vi "CRYUnary Curve.vi"(0 "Operand A":T2={"Name"="", "Curve"=[], "X data"=1, "Y data"=1, "Z data"=1, "X axis"=0, "Y axis"=1, "Z axis"=1, "X unit"="Hz", "Y unit"="", "Z unit"="deg.", "X dB ref"=1.0, "Y dB ref"=1.0, "Z dB ref"=1.0, "single val"=FALSE, "protected"=FALSE, "display X"=TRUE, "display Y"=TRUE, "display Z"=TRUE, "Test Info"="", "Step No."=0, "Plot Settings"={"Color"=0, "Interpolation"=0, "Point Style"=0, "Line Style"=0, "Point Color"=0, "Line Width"=0, "Bar Plot Style"=0, "Fill To"=0}, "AutoProtect"=FALSE} {"Z data" items=["dB", "Lin"]; "X data" items=["dB", "Lin"]; "Y data" items=["dB", "Lin"]; "Z dB ref" format="%.1f"; "Z axis" items=["Log", "Lin"]; "X dB ref" format="%.1f"; "X axis" items=["Log", "Lin"]; "Y axis" items=["Log", "Lin"]; "Y dB ref" format="%.1f"; "Curve"."z" format="%.2f"; "Curve"."y" format="%.2f"; "Curve"."x" format="%.2f"}, 1 "Type A":enum16{"Curves", "Values", "Results", "WFM"}(ring), 2 "All points":bool, 5 "A _axis mode":u16(slide) scale=0.0..2.0, 7 "Unary Operator":u16(ring) items=["Change Sign", "Reciprocal Value", "Absolute Value", "Square", "Square Root", "Exp", "Ln", "Unwarp Phase", "Group Delay", "FFT", "Inverse FFT"], 9 "Wave in":T1={"Waveform"={"X0"=0.0, "dX"=0.0, "Y"=[]}, "X data"=1, "Y data"=1, "Y axis"=1, "X unit"="s", "Y unit"="V", "Y dB ref"=1.0, "display Y"=TRUE, "display X"=TRUE, "Overload?"=FALSE, "Test Info"="", "Step No."=0, "Name"="", "protected"=FALSE, "Sqc history"=[], "Signal Channel ID"=0, "Plot Settings"={"Color"=0, "Interpolation"=0, "Point Style"=0, "Line Style"=0, "Point Color"=0, "Line Width"=0, "Bar Plot Style"=0, "Fill To"=0}, "AutoProtect"=FALSE} {"Y dB ref" format="%.1f"; "Y axis" items=["Log", "Lin"]; "Y data" items=["dB", "Lin"]; "X data" items=["dB", "Lin"]}, 11 "Search Items":string[](array[string]), 12 "Win Mode":u16(ring) items=["None", "Cosine Traper", "Exponential"], 13 "Smoothing Width":i32, 14 "Sampling Rate":dbl) -> (4 "Result":T2={"Name"="", "Curve"=[], "X data"=1, "Y data"=1, "Z data"=1, "X axis"=0, "Y axis"=1, "Z axis"=1, "X unit"="Hz", "Y unit"="", "Z unit"="deg.", "X dB ref"=1.0, "Y dB ref"=1.0, "Z dB ref"=1.0, "single val"=FALSE, "protected"=FALSE, "display X"=TRUE, "display Y"=TRUE, "display Z"=TRUE, "Test Info"="", "Step No."=0, "Plot Settings"={"Color"=0, "Interpolation"=0, "Point Style"=0, "Line Style"=0, "Point Color"=0, "Line Width"=0, "Bar Plot Style"=0, "Fill To"=0}, "AutoProtect"=FALSE} {"Z data" items=["dB", "Lin"]; "X data" items=["dB", "Lin"]; "Y data" items=["dB", "Lin"]; "Z dB ref" format="%.1f"; "Z axis" items=["Log", "Lin"]; "X dB ref" format="%.1f"; "X axis" items=["Log", "Lin"]; "Y axis" items=["Log", "Lin"]; "Y dB ref" format="%.1f"; "Curve"."z" format="%.2f"; "Curve"."y" format="%.2f"; "Curve"."x" format="%.2f"}, 6 "Type out":enum16{"Curves", "Values", "Results", "WFM"}(ring), 10 "Wave out":T1={"Waveform"={"X0"=0.0, "dX"=0.0, "Y"=[]}, "X data"=1, "Y data"=1, "Y axis"=1, "X unit"="s", "Y unit"="V", "Y dB ref"=1.0, "display Y"=TRUE, "display X"=TRUE, "Overload?"=FALSE, "Test Info"="", "Step No."=0, "Name"="", "protected"=FALSE, "Sqc history"=[], "Signal Channel ID"=0, "Plot Settings"={"Color"=0, "Interpolation"=0, "Point Style"=0, "Line Style"=0, "Point Color"=0, "Line Width"=0, "Bar Plot Style"=0, "Fill To"=0}, "AutoProtect"=FALSE} {"Y dB ref" format="%.1f"; "Y axis" items=["Log", "Lin"]; "Y data" items=["dB", "Lin"]; "X data" items=["dB", "Lin"]})   [LabVIEW 2013]
uses:
  Typedef Control/CRYData Cluster.ctl
  Typedef Control/CRYWaveform Cluster.ctl
  <vilib>/Analysis/4window.llb/Cosine Tapered Window (CDB).vi
  <vilib>/Analysis/4window.llb/Exponential Window (CDB).vi
  <vilib>/Analysis/2dsp.llb/Complex FFT.vi
  <vilib>/Analysis/2dsp.llb/Inverse Real FFT.vi
  CRYPost Processing Global.vi
  <vilib>/Analysis/NI_AALPro.lvlib
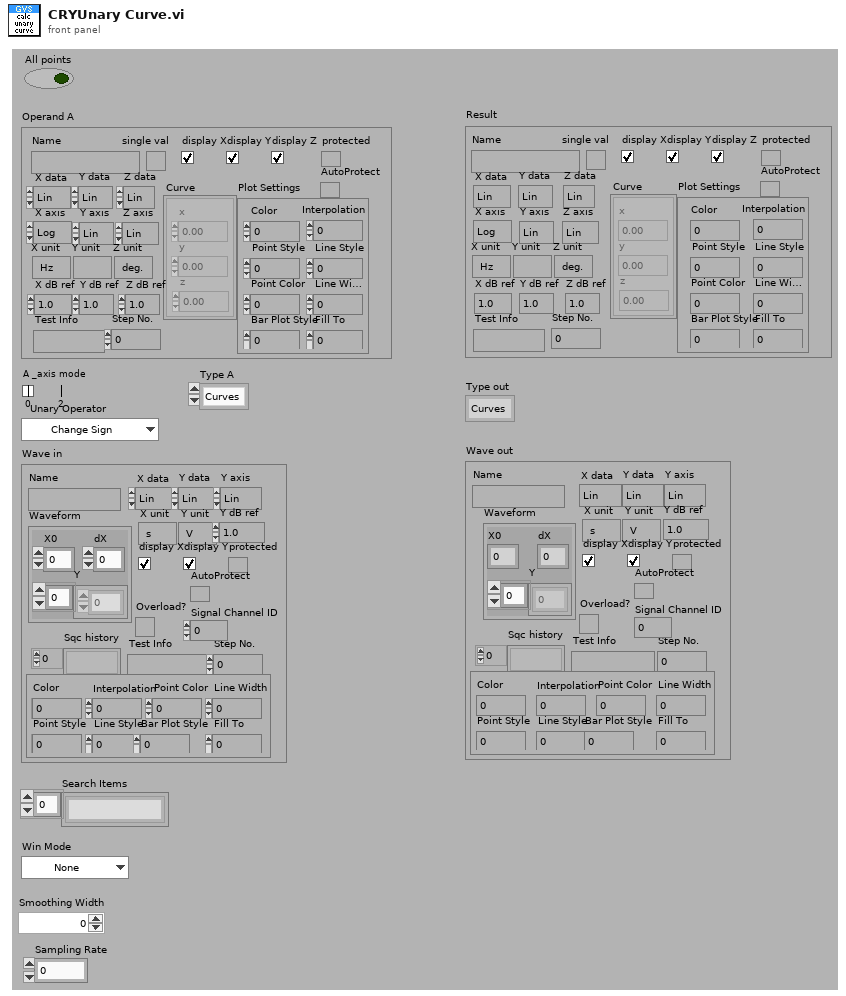
[diagram p1: front panel]
types:
  T1 = typedef "CRYWaveform Cluster.ctl" = cluster{"Waveform":cluster{"X0":dbl, "dX":dbl, "Y":sgl[]}, "X data":u16, "Y data":u16, "Y axis":u16, "X unit":string, "Y unit":string, "Y dB ref":dbl, "display Y":bool, "display X":bool, "Overload?":bool, "Test Info":string, "Step No.":i32, "Name":string, "protected":bool, "Sqc history":string[], "Signal Channel ID":i32, "Plot Settings":cluster{"Color":u32, "Interpolation":u8, "Point Style":u8, "Line Style":u8, "Point Color":u32, "Line Width":u8, "Bar Plot Style":u8, "Fill To":i16}, "AutoProtect":bool}
  T2 = typedef "CRYData Cluster.ctl" = cluster{"Name":string, "Curve":cluster{"x":dbl, "y":dbl, "z":dbl}[], "X data":u16, "Y data":u16, "Z data":u16, "X axis":u16, "Y axis":u16, "Z axis":u16, "X unit":string, "Y unit":string, "Z unit":string, "X dB ref":dbl, "Y dB ref":dbl, "Z dB ref":dbl, "single val":bool, "protected":bool, "display X":bool, "display Y":bool, "display Z":bool, "Test Info":string, "Step No.":i32, "Plot Settings":cluster{"Color":u32, "Interpolation":u8, "Point Style":u8, "Line Style":u8, "Point Color":u32, "Line Width":u8, "Bar Plot Style":u8, "Fill To":i16}, "AutoProtect":bool}
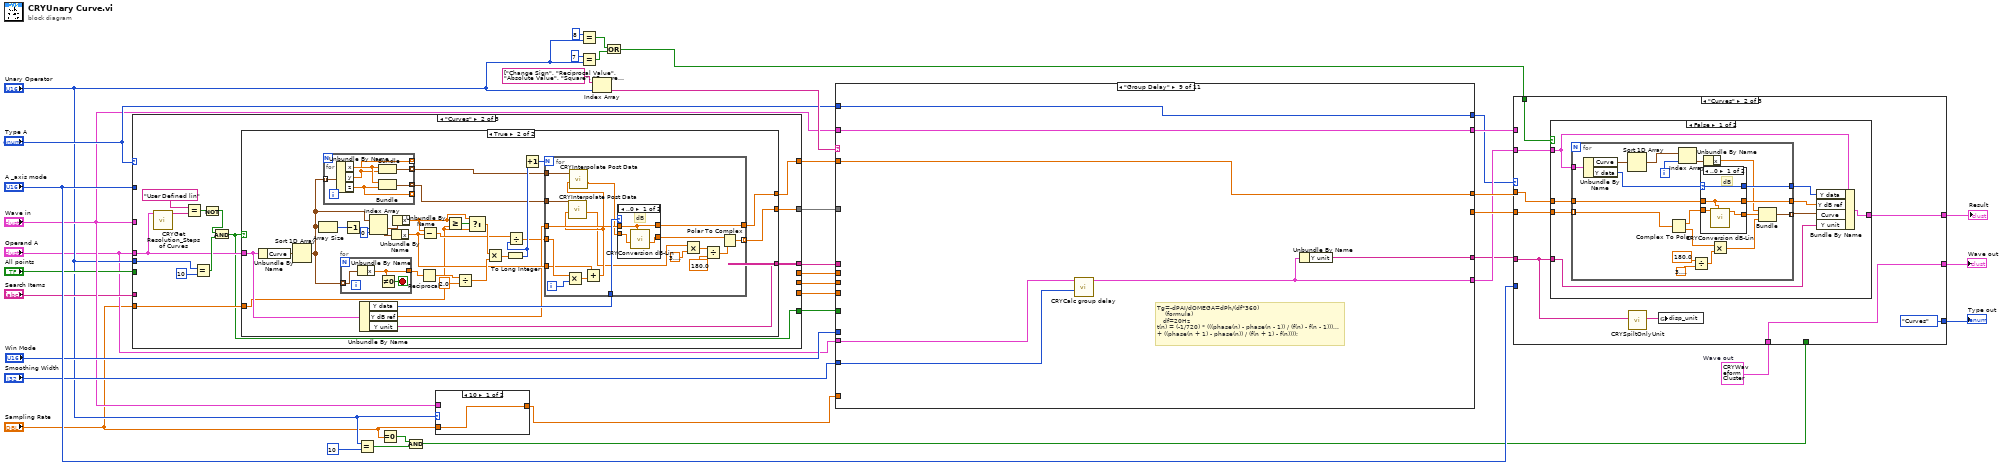
[diagram p0: block diagram]
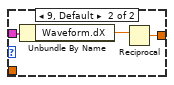
[diagram p2: hidden frame]
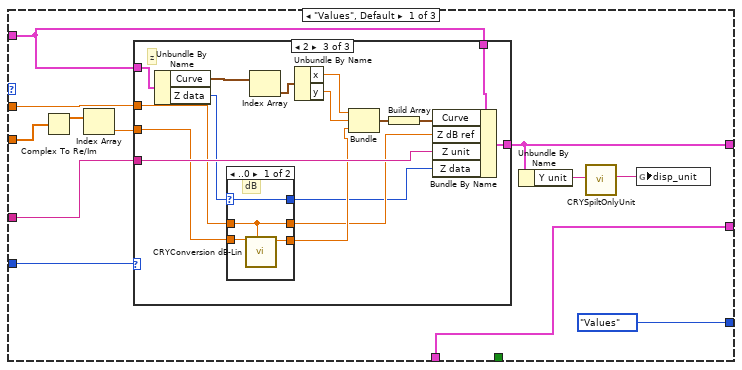
[diagram p3: hidden frame]
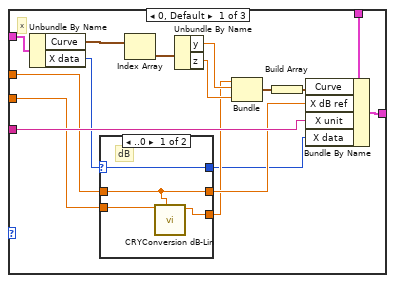
[diagram p4: hidden frame]
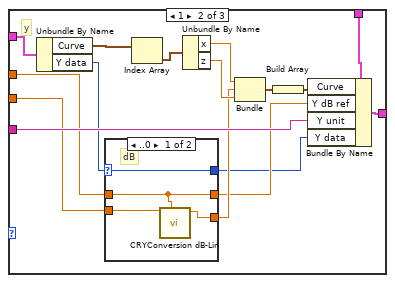
[diagram p6: hidden frame]
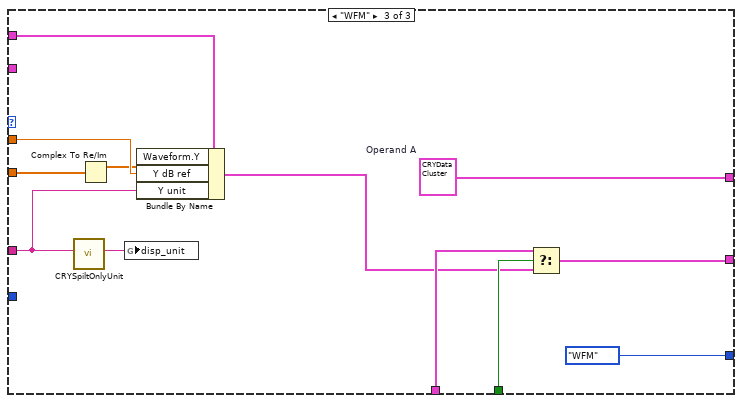
[diagram p11: hidden frame]
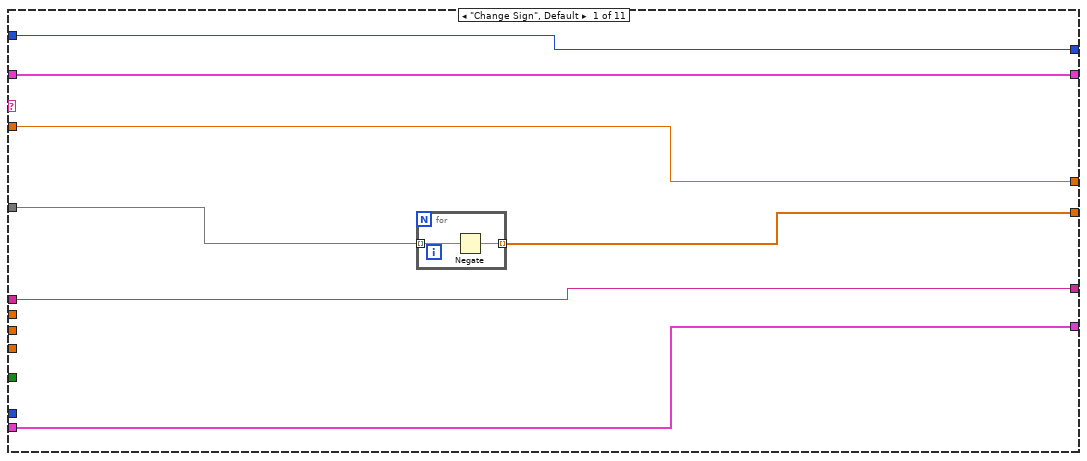
[diagram p12: hidden frame]
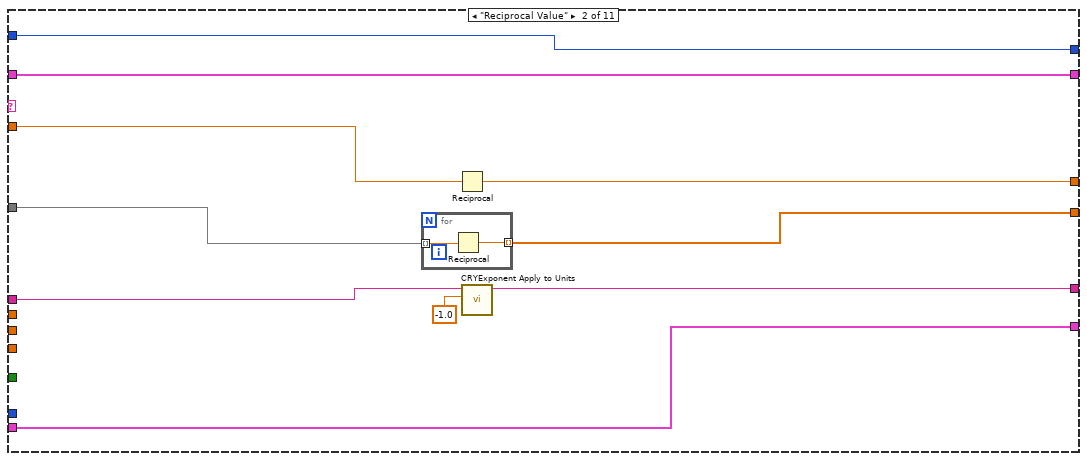
[diagram p13: hidden frame]
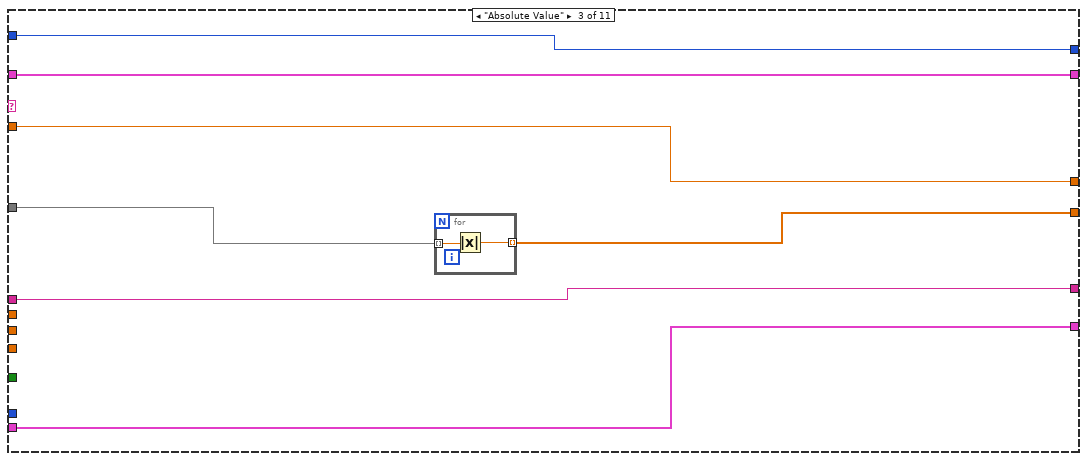
[diagram p14: hidden frame]
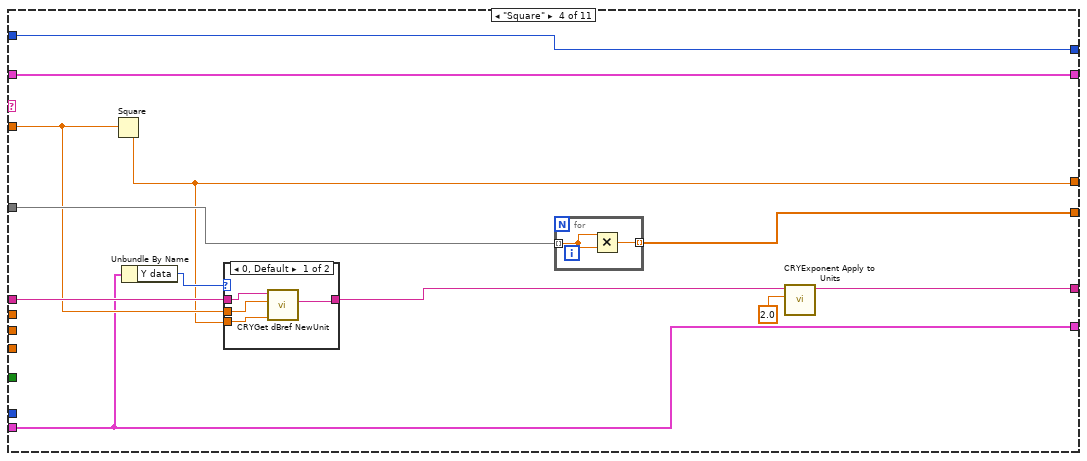
[diagram p15: hidden frame]
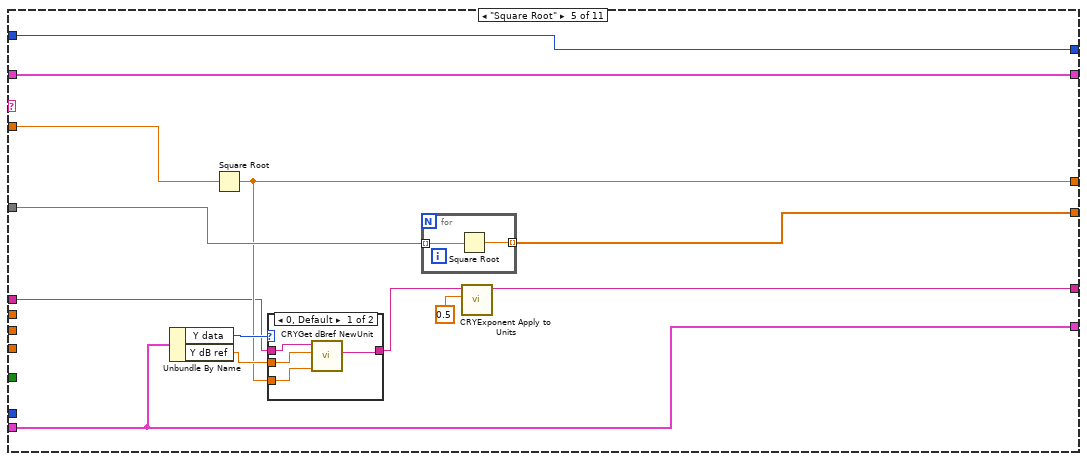
[diagram p17: hidden frame]
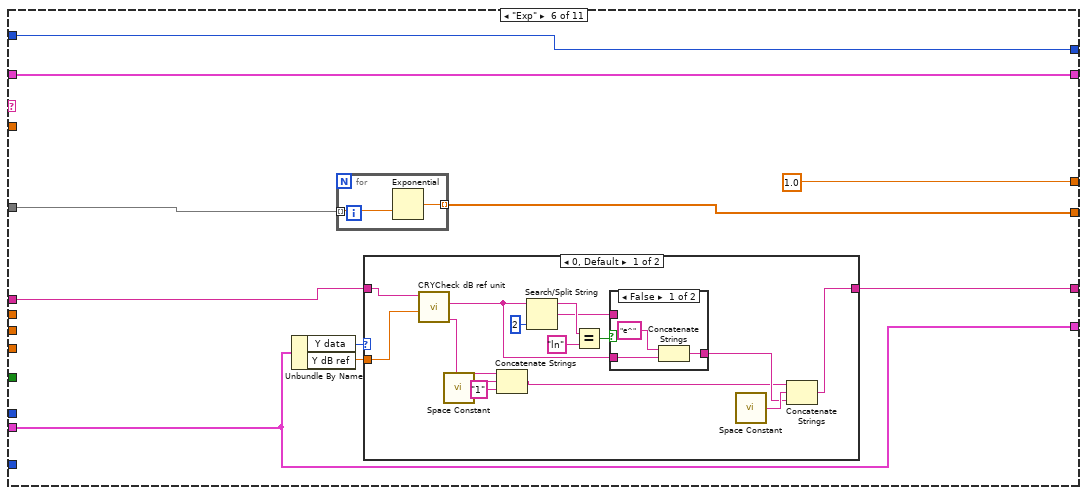
[diagram p19: hidden frame]
diagram:
  w5 = T1 {"Waveform"={"X0"=0.0, "dX"=0.0, "Y"=[]}, "X data"=1, "Y data"=1, "Y axis"=1, "X unit"="s", "Y unit"="V", "Y dB ref"=1.0, "display Y"=TRUE, "display X"=TRUE, "Overload?"=FALSE, "Test Info"="", "Step No."=0, "Name"="", "protected"=FALSE, "Sqc history"=[], "Signal Channel ID"=0, "Plot Settings"={"Color"=0, "Interpolation"=0, "Point Style"=0, "Line Style"=0, "Point Color"=0, "Line Width"=0, "Bar Plot Style"=0, "Fill To"=0}, "AutoProtect"=FALSE}  # Wave out
  n1 = case shown="\"Curves\"" "Type A" {
    tunnel: [w47 w100 w193] -> w12
    tunnel: [w46 w102 w201] -> w36
    tunnel: [w43 w101 w202] -> w37
    tunnel: "Operand A" -> [w44 w91 _]
    tunnel: "A _axis mode" -> [w45 _ _]
    tunnel: "Wave in" -> [_ _ w203]
    tunnel: "Search Items" -> [_ _ w196]
    tunnel: "All points" -> [_ _ w200]
    tunnel: [_ _ w195] -> w15
    tunnel: [_ _ w194] -> w14
    tunnel: [_ _ w192] -> w13
    tunnel: "Unary Operator" -> [_ w94 w191]
    tunnel: "Sampling Rate" -> [_ w99 _]
    tunnel: [_ w90 _] -> w2
    frame "Values", Default {
      n2 = case shown="0, Default" w45 {
        tunnel: w44 -> [w56 w68 w82]
        tunnel: [w48 w63 w76] -> w42
        tunnel: [w53 w67 w81] -> w46
        tunnel: [w49 w62 w77] -> w43
        frame 0, Default {
          # "x"
          n3 = Unbundle By Name(w56) -> ("X data"=w52:u16, "X dB ref"=w51:dbl, "Curve"=w55:cluster{"x":dbl, "y":dbl, "z":dbl}[], "X unit"=w53:string)
          n4 = Index Array(array=w55) -> (element=w54:cluster{"x":dbl, "y":dbl, "z":dbl})  [unwired: 1 in]
          n5 = Unbundle By Name(w54) -> ("x"=w50:dbl)
          n6 = case shown="1.." w52 {
            tunnel: w50 -> [w57 w61]
            tunnel: [w59 w61] -> w48
            tunnel: w51 -> [w58 w60]
            tunnel: [w58 w60] -> w49
            frame ..0 {
              # "dB"
              n7 = call "CRYConversion dB-Lin.vi"("dB ref."=w58, "Log In"=w57) -> ("Lin Out"=w59:dbl)  [unwired: 4 in, 3 out]
            }
            frame 1.. {
            }
          }
        }
        frame 1 {
          # "y"
          n8 = Unbundle By Name(w68) -> ("Y data"=w66:u16, "Y dB ref"=w64:dbl, "Curve"=w70:cluster{"x":dbl, "y":dbl, "z":dbl}[], "Y unit"=w67:string)
          n9 = Index Array(array=w70) -> (element=w69:cluster{"x":dbl, "y":dbl, "z":dbl})  [unwired: 1 in]
          n10 = Unbundle By Name(w69) -> ("y"=w65:dbl)
          n11 = case shown="1.." w66 {
            tunnel: w65 -> [w73 w75]
            tunnel: [w72 w75] -> w63
            tunnel: w64 -> [w71 w74]
            tunnel: [w71 w74] -> w62
            frame ..0 {
              # "dB"
              n12 = call "CRYConversion dB-Lin.vi"("dB ref."=w71, "Log In"=w73) -> ("Lin Out"=w72:dbl)  [unwired: 4 in, 3 out]
            }
            frame 1.. {
            }
          }
        }
        frame 2 {
          # "Z"
          n13 = Unbundle By Name(w82) -> ("Z data"=w80:u16, "Z dB ref"=w79:dbl, "Curve"=w84:cluster{"x":dbl, "y":dbl, "z":dbl}[], "Z unit"=w81:string)
          n14 = Index Array(array=w84) -> (element=w83:cluster{"x":dbl, "y":dbl, "z":dbl})  [unwired: 1 in]
          n15 = Unbundle By Name(w83) -> ("z"=w78:dbl)
          n16 = case shown="..0" w80 {
            tunnel: w78 -> [w86 w89]
            tunnel: [w87 w89] -> w76
            tunnel: w79 -> [w85 w88]
            tunnel: [w85 w88] -> w77
            frame ..0 {
              # "dB"
              n17 = call "CRYConversion dB-Lin.vi"("dB ref."=w85, "Log In"=w86) -> ("Lin Out"=w87:dbl)  [unwired: 4 in, 3 out]
            }
            frame 1.. {
            }
          }
        }
      }
      n18 = Polar To Complex(1:0.0 ("theta"), 2:w42) -> (0:w41:cdb)
      n19 = Build Array(w41) -> (w47:cdb[])
    }
    frame "Curves" {
      n20 = call "CRYGet Resolution_Steps of Curves.vi"("Curve In"=w91) -> ("Original Resolution Out"=w98:string)  [unwired: 9 in, 1 out]
      n21 = Equal?(x="User Defined lin", y=w98) -> (x = y?=w96:bool)
      n22 = Equal?(x=w94, y=u16 10) -> (x = y?=w92:bool)
      n23 = Not(x=w96) -> (.not. x?=w93:bool)
      n24 = And(x=w93, y=w92) -> (x .and. y?=w90:bool)
      n25 = case shown="True" w90 {
        tunnel: w91 -> [w110 w132]
        tunnel: [w109 w128] -> w102
        tunnel: [w108 w130] -> w101
        tunnel: [w107 w129] -> w100
        tunnel: w99 -> [_ w131]
        frame False {
          n26 = Unbundle By Name(w110) -> ("Y data"=w105:u16, "Y dB ref"=w104:dbl, "Curve"=w106:cluster{"x":dbl, "y":dbl, "z":dbl}[], "Y unit"=w109:string)
          n27 = Sort 1D Array(array=w106) -> (sorted array=w103:cluster{"x":dbl, "y":dbl, "z":dbl}[])
          n28 = for {
            tunnel: w103 -> [w122] mode=indexing
            tunnel: [w121] -> w107 mode=indexing
            tunnel: w105 -> [w120]
            tunnel: w104 -> [w113]
            tunnel: [w112] -> w108
            n29 = Unbundle By Name(w122) -> ("y"=w119:dbl, "z"=w114:dbl)  [unwired: 1 out]
            n30 = case shown="..0" w120 {
              tunnel: w119 -> [w124 w127]
              tunnel: [w125 w127] -> w111
              tunnel: w113 -> [w123 w126]
              tunnel: [w123 w126] -> w112
              frame ..0 {
                # "dB"
                n31 = call "CRYConversion dB-Lin.vi"("dB ref."=w123, "Log In"=w124) -> ("Lin Out"=w125:dbl)  [unwired: 4 in, 3 out]
              }
              frame 1.. {
              }
            }
            n32 = Multiply(x=w114, y=3.141592653589793) -> (x*y=w117:dbl)
            n33 = Divide(x=w117, y=180.0) -> (x/y=w118:dbl)
            n34 = Polar To Complex(1:w118, 2:w111) -> (0:w121:cdb)
          }
        }
        frame True {
          n35 = Unbundle By Name(w132) -> ("Curve"=w149:cluster{"x":dbl, "y":dbl, "z":dbl}[])
          n36 = Sort 1D Array(array=w149) -> (sorted array=w138:cluster{"x":dbl, "y":dbl, "z":dbl}[])
          n37 = Array Size(array=w138) -> (size(s)=w151:i32)
          n38 = for {
            tunnel: w138 -> [w165] mode=indexing
            tunnel: [w163] -> w137 mode=indexing
            tunnel: [w162] -> w136 mode=indexing
            tunnel: [w161] -> _ mode=indexing
            tunnel: [w160] -> _ mode=indexing
            n39 = Unbundle By Name(w165) -> ("x"=w164:dbl, "y"=w160:dbl, "z"=w161:dbl)
            n40 = Bundle("x"=w164, "y"=w160) -> (w163:cluster{"x":dbl, "y":dbl})  [unwired: 1 in]
            n41 = Bundle("x"=w164, "z"=w161) -> (w162:cluster{"x":dbl, "z":dbl})  [unwired: 1 in]
          }
          n42 = for {
            tunnel: w138 -> [w159] mode=indexing
            tunnel: [w157] -> w153
            stop <- w158 stop-if-true
            n43 = Unbundle By Name(w159) -> ("x"=w157:dbl)
            n44 = Not Equal To 0?(x=w157) -> (x != 0?=w158:bool)
          }
          n45 = Decrement(x=w151) -> (x-1=w150:i32)
          n46 = Unbundle By Name(w132) -> ("Y data"=w135:u16, "Y dB ref"=w134:dbl, "Y unit"=w128:string)
          n47 = Index Array(array=w138, index #1=w150, index #2=0 ("index")) -> (element #1=w152:cluster{"x":dbl, "y":dbl, "z":dbl}, element #2=w144:cluster{"x":dbl, "y":dbl, "z":dbl})
          n48 = Unbundle By Name(w144) -> ("x"=w139:dbl)
          n49 = Unbundle By Name(w152) -> ("x"=w143:dbl)
          n50 = Reciprocal(x=w153) -> (1/x=w148:dbl)
          n51 = Subtract(x=w143, y=w139) -> (x-y=w141:dbl)
          n52 = Greater Or Equal?(x=w143, y=w131) -> (x >= y?=w154:bool)
          n53 = Divide(x=w148, y=2.0) -> (x/y=w146:dbl)
          n54 = Select(t=w143, s=w154, f=w131) -> (s? t:f=w156:dbl)
          n55 = Multiply(x=w156, y=w146) -> (x*y=w155:dbl)
          n56 = To Long Integer(number=w155) -> (32bit integer=w140:i32)
          n57 = Divide(x=w141, y=w140) -> (x/y=w133:dbl)
          n58 = Increment(x=w140) -> (x+1=w142:i32)
          n59 = for {
            N: w142 -> [_]
            tunnel: w133 -> [w183]
            tunnel: w139 -> [w180]
            tunnel: w137 -> [w179]
            tunnel: w136 -> [w178]
            tunnel: w135 -> [w172]
            tunnel: w134 -> [w171]
            tunnel: [w170] -> w129 mode=indexing
            tunnel: [w169] -> w130
            i -> [w182]
            n60 = Multiply(x=w183, y=w182) -> (x*y=w181:dbl)
            n61 = Add(x=w180, y=w181) -> (x+y=w168:dbl)
            n62 = call "CRYInterpolate Post Data.vi"("X value"=w168, "Curve in"=w178) -> ("Y value"=w166:dbl)  [unwired: 9 in]
            n63 = call "CRYInterpolate Post Data.vi"("X value"=w168, "Curve in"=w179) -> ("Y value"=w167:dbl)  [unwired: 9 in]
            n64 = case shown="..0" w172 {
              tunnel: w167 -> [w185 w188]
              tunnel: [w186 w188] -> w173
              tunnel: w171 -> [w184 w187]
              tunnel: [w184 w187] -> w169
              frame ..0 {
                # "dB"
                n65 = call "CRYConversion dB-Lin.vi"("dB ref."=w184, "Log In"=w185) -> ("Lin Out"=w186:dbl)  [unwired: 4 in, 3 out]
              }
              frame 1.. {
              }
            }
            n66 = Multiply(x=w166, y=3.141592653589793) -> (x*y=w176:dbl)
            n67 = Divide(x=w176, y=180.0) -> (x/y=w177:dbl)
            n68 = Polar To Complex(1:w177, 2:w173) -> (0:w170:cdb)
          }
        }
      }
    }
    frame "WFM" {
      # "max"
      # "min"
      n69 = Unbundle By Name(w203) -> ("Y dB ref"=w202:dbl, "Waveform.Y"=w198:sgl[], "Y unit"=w201:string, "Waveform.X0"=w199:dbl, "Waveform.dX"=w197:dbl)
      n70 = Equal?(x=u16 9, y=w191) -> (x = y?=w189:bool)
      n71 = case shown="True" w189 {
        tunnel: w200 -> [_ w213]
        tunnel: w199 -> [_ w212]
        tunnel: w198 -> [w204 w211]
        tunnel: w197 -> [_ w210]
        tunnel: w196 -> [_ w209]
        tunnel: [_ w208] -> w195
        tunnel: [_ w207] -> w194
        tunnel: [w204 w206] -> w193
        tunnel: [_ w205] -> w192
        frame False {
        }
        frame True {
          n72 = case shown="False" w213 {
            tunnel: [w221 w235] -> w207
            tunnel: [w222 w238] -> w208
            tunnel: w212 -> [w225 w235]
            tunnel: w211 -> [w218 w236]
            tunnel: w210 -> [w220 w237]
            tunnel: w209 -> [w227 _]
            tunnel: [w215 w236] -> w206
            tunnel: [w214 w234] -> w205
            frame False {
              w228 = "%#p" ("format string")
              n73 = Index Array(array=w227) -> (element=w226:string)  [unwired: 1 in]
              n74 = Match Pattern(string=w226, regular expression="\\.\\.\\.") -> (before substring=w232:string, after substring=w231:string)  [unwired: 3 out]
              n75 = Scan Value(string=w231, format string=w228) -> (value=w229:dbl)  [unwired: 1 in, 1 out]
              n76 = Scan Value(string=w232, format string=w228) -> (value=w230:dbl)  [unwired: 1 in, 1 out]
              n77 = Max & Min(x=w230, y=w229) -> (max(x,y)=w222:dbl, min(x,y)=w221:dbl)
              n78 = Subtract(x=w221, y=w225) -> (x-y=w224:dbl)
              n79 = Divide(x=w224, y=w220) -> (x/y=w223:dbl)
              n80 = Subtract(x=w222, y=w221) -> (x-y=w214:dbl)
              n81 = To Long Integer(number=w223) -> (32bit integer=w217:i32)
              n82 = Divide(x=w214, y=w220) -> (x/y=w219:dbl)
              n83 = To Long Integer(number=w219) -> (32bit integer=w216:i32)
              n84 = Array Subset(array=w218, index=w217, length=w216) -> (w215:sgl[])
            }
            frame True {
              n85 = Array Size(array=w236) -> (size(s)=w239:i32)
              n86 = Multiply(x=w237, y=w239) -> (x*y=w234:dbl)
              n87 = Add(x=w235, y=w234) -> (x+y=w238:dbl)
            }
          }
        }
      }
    }
  }
  n88 = Equal?(x="Unary Operator", y=u16 10) -> (x = y?=w7:bool)
  n89 = Equal To 0?(x="Sampling Rate") -> (x = 0?=w8:bool)
  n90 = And(x=w8, y=w7) -> (x .and. y?=w6:bool)
  n91 = case shown="10" "Unary Operator" {
    tunnel: [w240 w242] -> w19
    tunnel: "Wave in" -> [_ w241]
    tunnel: "Sampling Rate" -> [w240 _]
    frame 10 {
    }
    frame 9, Default {
      n92 = Unbundle By Name(w241) -> ("Waveform.dX"=w243:dbl)
      n93 = Reciprocal(x=w243) -> (1/x=w242:dbl)
    }
  }
  n94 = Equal?(x=u16 8, y="Unary Operator") -> (x = y?=w22:bool)
  n95 = Equal?(x=u16 7, y="Unary Operator") -> (x = y?=w21:bool)
  n96 = Index Array(array=string[] ["Change Sign", "Reciprocal Value", "Absolute Value", "Square", "Square Root", "Exp", "Ln", "Unwarp Phase", "Group Delay", "FFT", "Inverse FFT"] ("Unary Op Name"), index="Unary Operator") -> (element=w39:string)
  n97 = Or(x=w22, y=w21) -> (x .or. y?=w20:bool)
  n98 = case shown="\"Group Delay\"" w39 {
    tunnel: w12 -> [w250 w262 w271 w285 w305 w322 w364 _ _ w431 w475]
    tunnel: [w249 w261 w270 w284 w304 w321 w363 _ _ w428 w479] -> w34
    tunnel: w36 -> [w247 w258 w268 w277 w294 w317 w361 w411 _ w442 _]
    tunnel: w37 -> [w248 w260 w269 w276 w303 _ _ w412 w427 _ w480]
    tunnel: [w248 w256 w269 w275 w295 1.0 1.0 w412 w427 w433 w480] -> w35
    tunnel: [w247 w257 w268 w282 w301 w320 w360 w411 w421 w437 w478] -> w1
    tunnel: "Win Mode" -> [_ _ _ _ _ _ _ _ _ w457 _]
    tunnel: "Operand A" -> [w246 w255 w267 w274 w298 w315 w357 w401 w426 w438 w477]
    tunnel: "Smoothing Width" -> [_ _ _ _ _ _ _ _ w425 _ _]
    tunnel: [w246 w255 w267 w274 w298 w315 w357 w400 w422 w439 w477] -> w33
    tunnel: w19 -> [_ _ _ _ _ _ _ _ _ w432 w476]
    tunnel: "Wave in" -> [w245 w254 w266 w280 w300 w314 w356 w410 w424 w436 w483]
    tunnel: [w245 w254 w266 w280 w300 w314 w356 w410 w424 w436 w481] -> w32
    tunnel: "Type A" -> [w244 w253 w265 w281 w299 w313 w355 w409 w423 _ _]
    tunnel: [w244 w253 w265 w281 w299 w313 w355 w409 w423 enum16{"Curves", "Values", "Results", "WFM"}."Curves" ("Type A") enum16{"Curves", "Values", "Results", "WFM"}."WFM" ("Type A")] -> w31
    tunnel: w15 -> [_ _ _ _ _ _ _ _ _ _ _]
    tunnel: w14 -> [_ _ _ _ _ _ _ _ _ _ _]
    tunnel: w13 -> [_ _ _ _ _ _ _ _ _ _ _]
    tunnel: w2 -> [_ _ _ _ _ _ _ _ _ _ w474]
    frame "Change Sign", Default {
      n99 = for {
        tunnel: w250 -> [w252] mode=indexing
        tunnel: [w251] -> w249 mode=indexing
        n100 = Negate(x=w252) -> (-x=w251:cdb)
      }
    }
    frame "Reciprocal Value" {
      n101 = for {
        tunnel: w262 -> [w264] mode=indexing
        tunnel: [w263] -> w261 mode=indexing
        n102 = Reciprocal(x=w264) -> (1/x=w263:cdb)
      }
      n103 = Reciprocal(x=w260) -> (1/x=w256:dbl)
      n104 = call "CRYExponent Apply to Units.vi"("Exponent to apply"=-1.0, "Unit in"=w258) -> ("Unit out"=w257:string)  [unwired: 9 out]
    }
    frame "Absolute Value" {
      n105 = for {
        tunnel: w271 -> [w273] mode=indexing
        tunnel: [w272] -> w270 mode=indexing
        n106 = Absolute Value(x=w273) -> (abs(x)=w272:dbl)
      }
    }
    frame "Square" {
      n107 = Square(x=w276) -> (x^2=w275:dbl)
      n108 = Unbundle By Name(w274) -> ("Y data"=w279:u16)
      n109 = case shown="0, Default" w279 {
        tunnel: [w286 w290] -> w278
        tunnel: w277 -> [w289 w290]
        tunnel: w276 -> [w288 _]
        tunnel: w275 -> [w287 _]
        frame 0, Default {
          n110 = call "CRYGet dBref NewUnit.vi"("New dB ref in"=w287, "Old dB ref in"=w288, "Unit in"=w289) -> ("Out New Unit"=w286:string)  [unwired: 8 in]
        }
        frame 1 {
        }
      }
      n111 = for {
        tunnel: w285 -> [w292] mode=indexing
        tunnel: [w291] -> w284 mode=indexing
        n112 = Multiply(x=w292, y=w292) -> (x*y=w291:cdb)
      }
      n113 = call "CRYExponent Apply to Units.vi"("Exponent to apply"=2.0, "Unit in"=w278) -> ("Unit out"=w282:string)  [unwired: 9 out]
    }
    frame "Square Root" {
      n114 = Unbundle By Name(w298) -> ("Y data"=w297:u16, "Y dB ref"=w296:dbl)
      n115 = Square Root(x=w303) -> (sqrt(x)=w295:dbl)
      n116 = case shown="0, Default" w297 {
        tunnel: [w306 w310] -> w293
        tunnel: w294 -> [w309 w310]
        tunnel: w296 -> [w308 _]
        tunnel: w295 -> [w307 _]
        frame 0, Default {
          n117 = call "CRYGet dBref NewUnit.vi"("New dB ref in"=w307, "Old dB ref in"=w308, "Unit in"=w309) -> ("Out New Unit"=w306:string)  [unwired: 8 in]
        }
        frame 1 {
        }
      }
      n118 = for {
        tunnel: w305 -> [w312] mode=indexing
        tunnel: [w311] -> w304 mode=indexing
        n119 = Square Root(x=w312) -> (sqrt(x)=w311:cdb)
      }
      n120 = call "CRYExponent Apply to Units.vi"("Exponent to apply"=0.5, "Unit in"=w293) -> ("Unit out"=w301:string)  [unwired: 9 out]
    }
    frame "Exp" {
      n121 = Unbundle By Name(w315) -> ("Y data"=w318:u16, "Y dB ref"=w316:dbl)
      n122 = for {
        tunnel: w322 -> [w354] mode=indexing
        tunnel: [w353] -> w321 mode=indexing
        n123 = Exponential(1:w354) -> (0:w353:cdb)
      }
      n124 = case shown="0, Default" w318 {
        tunnel: [w329 w348] -> w320
        tunnel: w317 -> [w330 w342]
        tunnel: w316 -> [w332 _]
        frame 0, Default {
          n125 = call "CRYCheck dB ref unit.vi"("dB ref in"=w332, "Unit in"=w330) -> ("dB re"=w326:string, "Lin unit out"=w331:string)  [unwired: 8 out]
          n126 = call <vilib>:"Space Constant.vi"() -> ("String"=w325:string)
          n127 = Concatenate Strings(w326, w325, "1" ("string")) -> (w323:string)
          n128 = Search/Split String(string=w331, offset (0)=2) -> (substring before match=w335:string, match + rest of string=w333:string)  [unwired: 2 out]
          n129 = Equal?(x=w335, y="ln") -> (x = y?=w334:bool)
          n130 = case shown="False" w334 {
            tunnel: w331 -> [w340 _]
            tunnel: [w338 w341] -> w327
            tunnel: w333 -> [_ w341]
            frame False {
              n131 = Concatenate Strings("e^", w340) -> (w338:string)
            }
            frame True {
            }
          }
          n132 = call <vilib>:"Space Constant.vi"() -> ("String"=w328:string)
          n133 = Concatenate Strings(w323, w328, w327) -> (w329:string)
        }
        frame 1 {
          n134 = Search/Split String(string=w342, offset (0)=2) -> (substring before match=w345:string, match + rest of string=w343:string)  [unwired: 2 out]
          n135 = Equal?(x=w345, y="ln") -> (x = y?=w344:bool)
          n136 = case shown="False" w344 {
            tunnel: w342 -> [w351 _]
            tunnel: [w349 w352] -> w348
            tunnel: w343 -> [_ w352]
            frame False {
              n137 = Concatenate Strings("e^", w351) -> (w349:string)
            }
            frame True {
            }
          }
        }
      }
    }
    frame "Ln" {
      # "Natural log:"
      n138 = Unbundle By Name(w357) -> ("Y data"=w359:u16, "Y dB ref"=w358:dbl)
      n139 = case shown="0, Default" w359 {
        tunnel: w361 -> [w370 w387]
        tunnel: [w367 w386] -> w360
        tunnel: w358 -> [w377 _]
        frame 0, Default {
          n140 = call "CRYCheck dB ref unit.vi"("dB ref in"=w377, "Unit in"=w370) -> ("dB ref N/dB ref N **?"=w366:bool, "Lin unit out"=w371:string)  [unwired: 8 out]
          n141 = case shown="False" w366 {
            tunnel: w371 -> [w380 _]
            tunnel: w370 -> [w379 w381]
            tunnel: [w378 w381] -> w365
            frame False {
              n142 = Search/Split String(string=w379, search string/char (-)=w380) -> (substring before match=w378:string)  [unwired: 3 out]
            }
            frame True {
            }
          }
          n143 = Search/Split String(string=w371, offset (0)=2) -> (substring before match=w374:string, match + rest of string=w372:string)  [unwired: 2 out]
          n144 = Equal?(x=w374, y="e^") -> (x = y?=w373:bool)
          n145 = case shown="False" w373 {
            tunnel: w371 -> [w384 _]
            tunnel: [w382 w385] -> w368
            tunnel: w372 -> [_ w385]
            frame False {
              n146 = Concatenate Strings("ln", w384) -> (w382:string)
            }
            frame True {
            }
          }
          n147 = call <vilib>:"Space Constant.vi"() -> ("String"=w369:string)
          n148 = Concatenate Strings(w365, w369, w368) -> (w367:string)
        }
        frame 1 {
          n149 = Search/Split String(string=w387, offset (0)=2) -> (substring before match=w390:string, match + rest of string=w388:string)  [unwired: 2 out]
          n150 = Equal?(x=w390, y="e^") -> (x = y?=w389:bool)
          n151 = case shown="False" w389 {
            tunnel: w387 -> [w395 _]
            tunnel: [w393 w396] -> w386
            tunnel: w388 -> [_ w396]
            frame False {
              n152 = Concatenate Strings("ln", w395) -> (w393:string)
            }
            frame True {
            }
          }
        }
      }
      n153 = for {
        tunnel: w364 -> [w398] mode=indexing
        tunnel: [w397] -> w363 mode=indexing
        n154 = Natural Logarithm(1:w398) -> (0:w397:cdb)
      }
    }
    frame "Unwarp Phase" {
      w408 = 2 items=["radian in, radian out", "radian in, degree out", "degree in, degree out", "degree in, radian out"] ("phase unit")
      n155 = Unbundle By Name(w401) -> ("Curve"=w407:cluster{"x":dbl, "y":dbl, "z":dbl}[])
      n156 = Sort 1D Array(array=w407) -> (sorted array=w399:cluster{"x":dbl, "y":dbl, "z":dbl}[])
      n157 = for {
        tunnel: w399 -> [w420] mode=indexing
        tunnel: [w419] -> w404 mode=indexing
        tunnel: [w418] -> w406 mode=indexing
        tunnel: [w417] -> w403 mode=indexing
        n158 = Unbundle By Name(w420) -> ("x"=w417:dbl, "y"=w419:dbl, "z"=w418:dbl)
      }
      n159 = call <vilib>:"Unwrap Phase.vi"("phase unit"=w408, "Phase"=w406) -> ("Unwrapped Phase"=w405:dbl[])  [unwired: 8 in, 1 out]
      n160 = for {
        tunnel: w405 -> [w414] mode=indexing
        tunnel: w404 -> [w415] mode=indexing
        tunnel: w403 -> [w416] mode=indexing
        tunnel: [w413] -> w402 mode=indexing
        n161 = Bundle("x"=w416, "y"=w415, w414) -> (w413:cluster{"x":dbl, "y":dbl, dbl})  [unwired: 1 in]
      }
      n162 = Bundle By Name(cluster=w401, "Curve"=w402) -> (w400:T2)
    }
    frame "Group Delay" {
      # "Tg=-dPAI/dOMEGA=dPh/(df*360)\n    (formula)\n   df=20Hz\nt(n) = (-1/720) * (((phase(n) - phase(n - 1)) / (f(n) - f(n - 1)))...\n+ ((phase(n + 1) - phase(n)) / (f(n + 1) - f(n))));"
      n163 = call "CRYCalc group delay.vi"("Smoothing Width"=w425, "Curve in"=w426) -> ("Curve out"=w422:T2)  [unwired: 9 out]
      n164 = Unbundle By Name(w422) -> ("Y unit"=w421:string)
    }
    frame "FFT" {
      w433 = 1.0 ("Y dB ref")
      n165 = case shown="0, Default" w457 {
        tunnel: w431 -> [w463 w465 w467]
        tunnel: [w463 w464 w466] -> w430
        frame 0, Default {
        }
        frame 1 {
          n166 = call-poly <vilib>:"Cosine Tapered Window.vi"("X"=w465) -> ("Windowed X"=w464:cdb[])  [unwired: 1 in, 9 out]
        }
        frame 2 {
          n167 = call-poly <vilib>:"Exponential Window.vi"("X"=w467) -> ("Windowed X"=w466:cdb[])  [unwired: 1 in, 1 out]
        }
      }
      n168 = call-poly <vilib>:"FFT.vi"("X"=w430) -> ("FFT {X}"=w429:cdb[])  [unwired: 2 in, 8 out]
      n169 = Array Size(array=w429) -> (size(s)=w452:i32)
      n170 = Quotient & Remainder(x=w452, y=2) -> (x-y*floor(x/y)=w455:i32, floor(x/y)=w454:i32)
      n171 = Add(x=w455, y=w454) -> (x+y=w453:i32)
      n172 = Array Subset(array=w429, length=w453) -> (w428:cdb[])  [unwired: 1 in]
      n173 = Array Size(array=w428) -> (size(s)=w441:i32)
      n174 = Divide(x=w432, y=2.0) -> (x/y=w446:dbl)
      n175 = Divide(x=w446, y=w441) -> (x/y=w445:dbl)
      n176 = for {
        N: w441 -> [_]
        tunnel: w445 -> [w461]
        tunnel: [w459] -> w440 mode=indexing
        tunnel: cluster{"x":dbl, "y":dbl, "z":dbl} {"x"=0.0, "y"=0.0, "z"=0.0} ("element") -> [w458]
        i -> [w462]
        n177 = Multiply(x=w461, y=w462) -> (x*y=w460:dbl)
        n178 = Bundle By Name(cluster=w458, "x"=w460) -> (w459:cluster{"x":dbl, "y":dbl, "z":dbl})
      }
      n179 = Format Value(format string="%#p", value (0)=w433) -> (output string=w449:string)  [unwired: 1 in]
      n180 = Bundle By Name(cluster=w438, "Curve"=w440, "X unit"="Hz", "Y data"=u16 0) -> (w439:T2)
      n181 = call <vilib>:"Space Constant.vi"() -> ("String"=w450:string)
      n182 = Concatenate Strings("dB re" ("Y unit"), w450, w449, w450, w442) -> (w437:string)
    }
    frame "Inverse FFT" {
      w517 = "s" ("X unit")
      n183 = Array Size(array=w475) -> (size(s)=w507:i32)
      n184 = Unbundle By Name(w477) -> ("Curve"=w497:cluster{"x":dbl, "y":dbl, "z":dbl}[])
      n185 = Reverse 1D Array(array=w475) -> (reversed array=w505:cdb[])
      n186 = Decrement(x=w507) -> (x-1=w506:i32)
      n187 = Sort 1D Array(array=w497) -> (sorted array=w493:cluster{"x":dbl, "y":dbl, "z":dbl}[])
      n188 = Delete From Array(array=w505, index=w506) -> (array with subset deleted=w504:cdb[])  [unwired: 1 in, 1 out]
      n189 = Build Array (concatenate)(w475, w504) -> (w498:cdb[])
      n190 = Array Size(array=w493) -> (size(s)=w495:i32)
      n191 = call-poly <vilib>:"Inverse FFT.vi"("FFT {X}"=w498) -> ("X"=w486:dbl[])  [unwired: 1 in, 9 out]
      n192 = Index Array(array=w493, index #1=1 ("index"), index #2=0 ("index")) -> (element #1=w471:cluster{"x":dbl, "y":dbl, "z":dbl}, element #2=w470:cluster{"x":dbl, "y":dbl, "z":dbl})
      n193 = Decrement(x=w495) -> (x-1=w496:i32)
      n194 = Index Array(array=w493, index=w496) -> (element=w494:cluster{"x":dbl, "y":dbl, "z":dbl})
      n195 = Unbundle By Name(w471) -> ("x"=w469:dbl)
      n196 = Unbundle By Name(w470) -> ("x"=w468:dbl)
      n197 = Unbundle By Name(w494) -> ("x"=w490:dbl)
      n198 = Subtract(x=w469, y=w468) -> (x-y=w492:dbl)
      n199 = Reciprocal(x=w492) -> (1/x=w487:dbl)
      n200 = Greater Or Equal?(x=w490, y=w476) -> (x >= y?=w491:bool)
      n201 = Equal To 0?(x=w476) -> (x = 0?=w503:bool)
      n202 = Select(t=w490, s=w491, f=w476) -> (s? t:f=w488:dbl)
      n203 = Multiply(x=w488, y=w487) -> (x*y=w489:dbl)
      n204 = To Long Integer(number=w489) -> (32bit integer=w484:i32)
      n205 = case shown="False" w474 {
        tunnel: w486 -> [w525 w531]
        tunnel: [w523 w531] -> w485
        tunnel: w484 -> [w521 _]
        frame False {
          n206 = Array Size(array=w525) -> (size(s)=w522:i32)
          n207 = Divide(x=w522, y=w521) -> (x/y=w524:dbl)
          n208 = for {
            N: w521 -> [_]
            tunnel: w525 -> [w527]
            tunnel: w524 -> [w529]
            tunnel: [w526] -> w523 mode=indexing
            i -> [w530]
            n209 = Multiply(x=w530, y=w529) -> (x*y=w528:dbl)
            n210 = Interpolate 1D Array(1:w528, 2:w527) -> (0:w526:dbl)
          }
        }
        frame True {
        }
      }
      n211 = Select(t=1.0, s=w503, f=w476) -> (s? t:f=w501:dbl)
      n212 = Unbundle By Name(w477) -> ("Y data"=w520:u16)
      n213 = Array Size(array=w485) -> (size(s)=w512:i32)
      n214 = Reciprocal(x=w501) -> (1/x=w500:dbl)
      n215 = case shown="0, Default" w520 {
        tunnel: w477 -> [w533 w537]
        tunnel: [w532 w536] -> w518
        frame 0, Default {
          n216 = Unbundle By Name(w533) -> ("Y unit"=w535:string, "Y dB ref"=w534:dbl)
          n217 = call "CRYCheck dB ref unit.vi"("dB ref in"=w534, "Unit in"=w535) -> ("Lin unit out"=w532:string)  [unwired: 6 in, 3 out]
        }
        frame 1 {
          n218 = Unbundle By Name(w537) -> ("Y unit"=w536:string)
        }
      }
      n219 = Quotient & Remainder(x=w512, y=2) -> (x-y*floor(x/y)=w515:i32, floor(x/y)=w514:i32)
      n220 = Add(x=w515, y=w514) -> (x+y=w513:i32)
      n221 = Subtract(x=w512, y=w513) -> (x-y=w509:i32)
      n222 = Multiply(x=w509, y=w500) -> (x*y=w508:dbl)
      n223 = Array Subset(array=w485, index=w513, length=w509) -> (w511:dbl[])
      n224 = Array Subset(array=w485, length=w513) -> (w510:dbl[])  [unwired: 1 in]
      n225 = Negate(x=w508) -> (-x=w499:dbl)
      n226 = Concatenate Strings(w518, "/" ("string"), w517) -> (w478:string)
      n227 = Build Array (concatenate)(w511, w510) -> (w479:dbl[])
      n228 = Bundle By Name(cluster=w483, "X unit"=w517, "Waveform.dX"=w500, "Waveform.X0"=w499) -> (w481:T1)
    }
  }
  n229 = case shown="\"Curves\"" w31 {
    tunnel: w34 -> [w545 w627 w671]
    tunnel: w33 -> [w543 w624 _]
    tunnel: w35 -> [w549 w626 w670]
    tunnel: w1 -> [w548 w619 w664]
    tunnel: [w540 w625 w674] -> w11
    tunnel: "A _axis mode" -> [w547 _ _]
    tunnel: [enum16{"Curves", "Values", "Results", "WFM"}."Values" ("Type In") enum16{"Curves", "Values", "Results", "WFM"}."Curves" ("Type In") enum16{"Curves", "Values", "Results", "WFM"}."WFM" ("Type In")] -> w25
    tunnel: [w541 w622 w665] -> w26
    tunnel: w32 -> [_ _ w672]
    tunnel: w20 -> [_ w621 _]
    tunnel: w6 -> [_ _ w668]
    tunnel: w5 -> [w541 w622 w667]
    frame "Values", Default {
      n230 = Complex To Re/Im(x + iy=w545) -> (x=w546:dbl[])  [unwired: 1 out]
      n231 = Index Array(array=w546) -> (element=w544:dbl)  [unwired: 1 in]
      n232 = case shown="2" w547 {
        tunnel: w544 -> [w552 w576 w599]
        tunnel: w543 -> [w561 w584 w607]
        tunnel: w549 -> [w554 w577 w600]
        tunnel: w548 -> [w562 w582 w608]
        tunnel: [w560 w583 w606] -> w540
        tunnel: w543 -> [w557 w580 w603]
        frame 0, Default {
          # "x"
          n233 = Unbundle By Name(w557) -> ("Curve"=w558:cluster{"x":dbl, "y":dbl, "z":dbl}[], "X data"=w555:u16)
          n234 = case shown="..0" w555 {
            selector: w555 -> [w568 w570]
            tunnel: w552 -> [w569 w572]
            tunnel: [w566 w572] -> w551
            tunnel: w554 -> [w567 w571]
            tunnel: [w567 w571] -> w553
            tunnel: [w568 w570] -> w550
            frame ..0 {
              # "dB"
              n235 = call "CRYConversion dB-Lin.vi"("dB ref."=w567, "Lin In"=w569) -> ("Log Out"=w566:dbl)  [unwired: 4 in, 3 out]
            }
            frame 1.. {
            }
          }
          n236 = Index Array(array=w558) -> (element=w556:cluster{"x":dbl, "y":dbl, "z":dbl})  [unwired: 1 in]
          n237 = Unbundle By Name(w556) -> ("y"=w559:dbl, "z"=w565:dbl)
          n238 = Bundle("Numeric"=w551, "y"=w559, "z"=w565) -> (w564:cluster{"Numeric":dbl, "y":dbl, "z":dbl})  [unwired: 1 out]
          n239 = Build Array(w564) -> (w563:cluster{"Numeric":dbl, "y":dbl, "z":dbl}[])
          n240 = Bundle By Name(cluster=w561, "Curve"=w563, "X dB ref"=w553, "X unit"=w562, "X data"=w550) -> (w560:T2)
        }
        frame 1 {
          # "y"
          n241 = Unbundle By Name(w580) -> ("Curve"=w581:cluster{"x":dbl, "y":dbl, "z":dbl}[], "Y data"=w578:u16)
          n242 = case shown="..0" w578 {
            selector: w578 -> [w591 w593]
            tunnel: w576 -> [w592 w595]
            tunnel: [w590 w595] -> w575
            tunnel: w577 -> [w589 w594]
            tunnel: [w589 w594] -> w574
            tunnel: [w591 w593] -> w573
            frame ..0 {
              # "dB"
              n243 = call "CRYConversion dB-Lin.vi"("dB ref."=w589, "Lin In"=w592) -> ("Log Out"=w590:dbl)  [unwired: 4 in, 3 out]
            }
            frame 1.. {
            }
          }
          n244 = Index Array(array=w581) -> (element=w579:cluster{"x":dbl, "y":dbl, "z":dbl})  [unwired: 1 in]
          n245 = Unbundle By Name(w579) -> ("x"=w588:dbl, "z"=w587:dbl)
          n246 = Bundle("x"=w588, "Numeric"=w575, "z"=w587) -> (w586:cluster{"x":dbl, "Numeric":dbl, "z":dbl})  [unwired: 1 out]
          n247 = Build Array(w586) -> (w585:cluster{"x":dbl, "Numeric":dbl, "z":dbl}[])
          n248 = Bundle By Name(cluster=w584, "Curve"=w585, "Y dB ref"=w574, "Y unit"=w582, "Y data"=w573) -> (w583:T2)
        }
        frame 2 {
          # "z"
          n249 = Unbundle By Name(w603) -> ("Curve"=w604:cluster{"x":dbl, "y":dbl, "z":dbl}[], "Z data"=w601:u16)
          n250 = case shown="..0" w601 {
            selector: w601 -> [w614 w616]
            tunnel: w599 -> [w615 w618]
            tunnel: [w613 w618] -> w598
            tunnel: w600 -> [w612 w617]
            tunnel: [w612 w617] -> w597
            tunnel: [w614 w616] -> w596
            frame ..0 {
              # "dB"
              n251 = call "CRYConversion dB-Lin.vi"("dB ref."=w612, "Lin In"=w615) -> ("Log Out"=w613:dbl)  [unwired: 4 in, 3 out]
            }
            frame 1.. {
            }
          }
          n252 = Index Array(array=w604) -> (element=w602:cluster{"x":dbl, "y":dbl, "z":dbl})  [unwired: 1 in]
          n253 = Unbundle By Name(w602) -> ("x"=w611:dbl, "y"=w605:dbl)
          n254 = Bundle("x"=w611, "y"=w605, "Numeric"=w598) -> (w610:cluster{"x":dbl, "y":dbl, "Numeric":dbl})  [unwired: 1 out]
          n255 = Build Array(w610) -> (w609:cluster{"x":dbl, "y":dbl, "Numeric":dbl}[])
          n256 = Bundle By Name(cluster=w607, "Curve"=w609, "Z dB ref"=w597, "Z unit"=w608, "Z data"=w596) -> (w606:T2)
        }
      }
      n257 = Unbundle By Name(w540) -> ("Y unit"=w538:string)
      n258 = call "CRYSpiltOnlyUnit.vi"("In Unit String"=w538) -> ("Out Unit String"=w539:string)  [unwired: 10 in]
      n259 = global write "CRYPost Processing Global.vi" "disp_unit"(w539) -> ()
    }
    frame "Curves" {
      n260 = case shown="False" w621 {
        tunnel: w627 -> [w635 _]
        tunnel: w626 -> [w634 _]
        tunnel: w619 -> [w633 _]
        tunnel: [w629 w662] -> w625
        tunnel: w624 -> [w628 w662]
        frame False {
          n261 = for {
            tunnel: [w654] -> w630 mode=indexing
            tunnel: w635 -> [w653] mode=indexing
            tunnel: w628 -> [w644]
            tunnel: w634 -> [w643]
            tunnel: [w642] -> w632
            tunnel: [w640] -> w631
            i -> [w639]
            n262 = Unbundle By Name(w644) -> ("Curve"=w645:cluster{"x":dbl, "y":dbl, "z":dbl}[], "Y data"=w641:u16)
            n263 = Sort 1D Array(array=w645) -> (sorted array=w636:cluster{"x":dbl, "y":dbl, "z":dbl}[])
            n264 = Complex To Polar(r * e^(i*theta)=w653) -> (r=w648:dbl, theta=w652:dbl)
            n265 = Index Array(array=w636, index=w639) -> (element=w646:cluster{"x":dbl, "y":dbl, "z":dbl})
            n266 = Divide(x=180.0, y=3.141592653589793) -> (x/y=w651:dbl)
            n267 = case shown="..0" w641 {
              selector: w641 -> [w657 w659]
              tunnel: w648 -> [w658 w661]
              tunnel: [w656 w661] -> w637
              tunnel: w643 -> [w655 w660]
              tunnel: [w655 w660] -> w642
              tunnel: [w657 w659] -> w640
              frame ..0 {
                # "dB"
                n268 = call "CRYConversion dB-Lin.vi"("dB ref."=w655, "Lin In"=w658) -> ("Log Out"=w656:dbl)  [unwired: 4 in, 3 out]
              }
              frame 1.. {
              }
            }
            n269 = Unbundle By Name(w646) -> ("x"=w638:dbl)
            n270 = Multiply(x=w652, y=w651) -> (x*y=w647:dbl)
            n271 = Bundle("x"=w638, "Log Out"=w637, w647) -> (w654:cluster{"x":dbl, "Log Out":dbl, dbl})  [unwired: 1 out]
          }
          n272 = Bundle By Name(cluster=w628, "Y data"=w631, "Y dB ref"=w632, "Curve"=w630, "Y unit"=w633) -> (w629:T2)
        }
        frame True {
        }
      }
      n273 = call "CRYSpiltOnlyUnit.vi"("In Unit String"=w619) -> ("Out Unit String"=w620:string)  [unwired: 10 in]
      n274 = global write "CRYPost Processing Global.vi" "disp_unit"(w620) -> ()
    }
    frame "WFM" {
      w674 = T2 {"Name"="", "Curve"=[], "X data"=1, "Y data"=1, "Z data"=1, "X axis"=0, "Y axis"=1, "Z axis"=1, "X unit"="Hz", "Y unit"="", "Z unit"="deg.", "X dB ref"=1.0, "Y dB ref"=1.0, "Z dB ref"=1.0, "single val"=FALSE, "protected"=FALSE, "display X"=TRUE, "display Y"=TRUE, "display Z"=TRUE, "Test Info"="", "Step No."=0, "Plot Settings"={"Color"=0, "Interpolation"=0, "Point Style"=0, "Line Style"=0, "Point Color"=0, "Line Width"=0, "Bar Plot Style"=0, "Fill To"=0}, "AutoProtect"=FALSE}  # Operand A
      n275 = call "CRYSpiltOnlyUnit.vi"("In Unit String"=w664) -> ("Out Unit String"=w663:string)  [unwired: 10 in]
      n276 = Complex To Re/Im(x + iy=w671) -> (x=w669:dbl[])  [unwired: 1 out]
      n277 = global write "CRYPost Processing Global.vi" "disp_unit"(w663) -> ()
      n278 = Bundle By Name(cluster=w672, "Waveform.Y"=w669, "Y dB ref"=w670, "Y unit"=w664) -> (w666:T1)
      n279 = Select(t=w667, s=w668, f=w666) -> (s? t:f=w665:T1)
    }
  }
  "Wave out" <- w26
  "Type out" <- w25
  "Result" <- w11
